vi "DEMO_Queue.vi"() -> ()   [LabVIEW 2018]
uses:
  DataPacker/DataStructures/GEM_BANK_CLUSTER_typedef.ctl
  DataPacker/DataStructures/GEM_DATA_cluster_typedef.ctl
  74751eb5-3986-46dd-b866-627731c09b6a.vi
  26fe34b5-c06c-455e-b018-4450bbc8faa2.vi
  74751eb5-3986-46dd-b866-627731c09b6a.vi/85c5be8d-80e5-4349-a72a-c74fdeb0c9bb.vi
  26fe34b5-c06c-455e-b018-4450bbc8faa2.vi/8747a64a-e124-4754-8124-08412923ccb0.vi
panel:
  in  "Request Debug Mode":bool
  in  "MIDAS Sever Port":u16=12345
  in  "MIDAS Server":string="my_midas_server.domain"
  out "RUNNO":i32
  in  "y":i32=2147483647
  in  "stop":bool
  out "# pending insert":i32
  out "# pending remove":i32
  out "# elements in queue":i32
  in  "Int entries to log":i32
  in  "IntState array":u32[](array[numeric])=[1, 2, 3, 4, 5, 6, 7, 8, 9, 10]
  in  "Entries to log":i32
  in  "Temperature array":dbl[](array[numeric])=[0.1, 0.2, 0.3, 0.4, 0.5, 0.6, 0.7, 0.8, 0.9, 1.0]
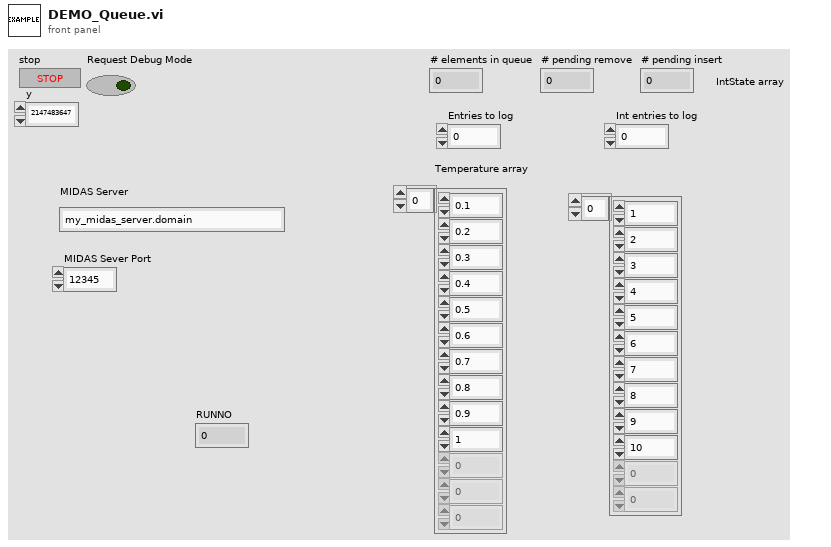
[diagram p1: front panel]
types:
  T1 = typedef "GEM_BANK_CLUSTER_typedef.ctl" = cluster{"Category":string, "Variable Name":string, "Equipment description":string, "History Settings":u16, "Period to update history plots":u16, "GEM_DATA Cluster":T2}
  T2 = typedef "GEM_DATA_cluster_typedef.ctl" = cluster{"DataType":string, "Formatted Data":u8[], "data byte order (Little Endian prefered)":enum16{"big-endian, network order", "native, host order", "little-endian"}}
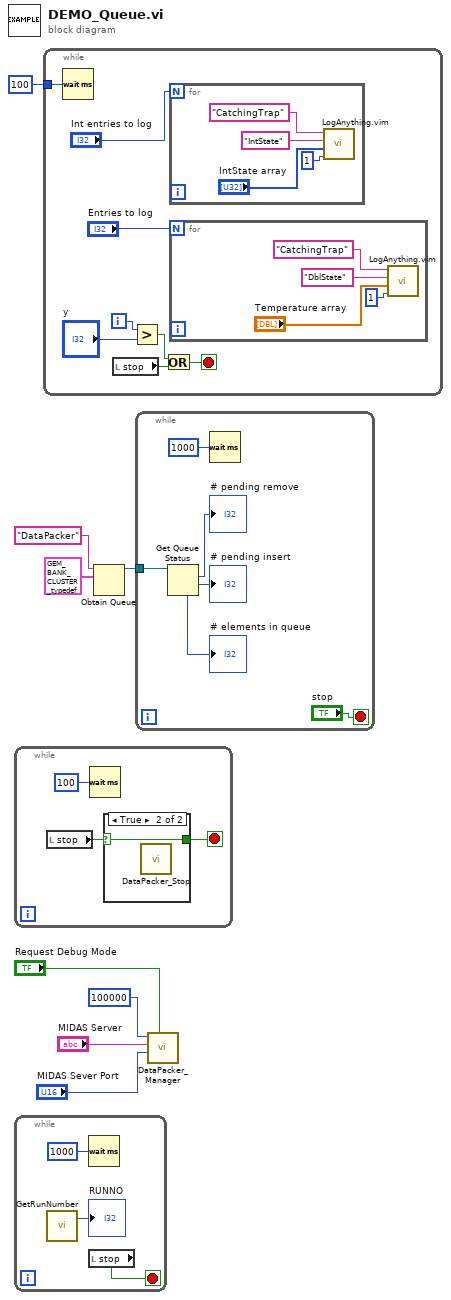
[diagram p0: block diagram]
diagram:
  n1 = while {
    stop <- w10 stop-if-true
    n2 = local read "stop"() -> (w9:bool)
    n3 = Wait (ms)(milliseconds to wait=u32 100) -> ()  [unwired: 1 out]
    n4 = case shown="True" w9 {
      selector: w9 -> [w12 w13]
      tunnel: [w12 w13] -> w10
      frame False {
      }
      frame True {
        n5 = call "DataPacker_Stop.vi"() -> ()  [unwired: 12 in]
      }
    }
  }
  n6 = while {
    stop <- w14 stop-if-true
    n7 = call "GetRunNumber.vi"() -> ("RunNumber"=→"RUNNO":i32)  [unwired: 2 in, 1 out]
    n8 = Wait (ms)(milliseconds to wait=u32 1000) -> ()  [unwired: 1 out]
    n9 = local read "stop"() -> (w14:bool)
  }
  n10 = while {
    tunnel: i64 100 ("Period") -> [w17]
    i -> [w18]
    stop <- w19 stop-if-true
    n11 = Wait (ms)(milliseconds to wait=w17) -> ()  [unwired: 1 out]
    n12 = local read "stop"() -> (w20:bool)
    n13 = Greater?(x=w18, y="y") -> (0:w21:bool)
    n14 = Or(x=w21, y=w20) -> (x .or. y?=w19:bool)
    n15 = for {
      N: "Int entries to log" -> [_]
      n16 = call "LogAnything.vim"("Period to update history plots (seconds)\nUnset (65535) = Use MIDAS default in ODB\n0 = Record but do not put in histories"=1 ("Rate to update history plots"), "Array"="IntState array", "Var Name"="IntState", "Category"="CatchingTrap") -> ()  [unwired: 3 in, 1 out]
    }
    n17 = for {
      N: "Entries to log" -> [_]
      n18 = call "LogAnything.vim"("Period to update history plots (seconds)\nUnset (65535) = Use MIDAS default in ODB\n0 = Record but do not put in histories"=1 ("Rate to update history plots"), "Array"="Temperature array", "Var Name"="DblState", "Category"="CatchingTrap") -> ()  [unwired: 3 in, 1 out]
    }
  }
  n19 = Obtain Queue(name (unnamed)="DataPacker", element data type=T1 {"Category"="", "Variable Name"="", "Equipment description"="", "History Settings"=0, "Period to update history plots"=0, "GEM_DATA Cluster"={"DataType"="", "Formatted Data"=[], "data byte order (Little Endian prefered)"=enum."big-endian, network order"}} ("output cluster")) -> (queue out=w7:refnum<queue>)  [unwired: 3 in, 2 out]
  n20 = while {
    tunnel: w7 -> [w38]
    stop <- "stop" stop-if-true
    n21 = Get Queue Status(queue=w38) -> (# pending remove=→"# pending remove":i32, # pending insert=→"# pending insert":i32, # elements in queue=→"# elements in queue":i32)  [unwired: 2 in, 5 out]
    n22 = Wait (ms)(milliseconds to wait=u32 1000) -> ()  [unwired: 1 out]
  }
  n23 = call "DataPacker_Manager.vi"("Request Debug Mode"="Request Debug Mode", "MIDAS Sever Port"="MIDAS Sever Port", "MIDAS Server"="MIDAS Server", "Override Max Event size (Data rate kb/s). Use MIDAS Default = 0"=u32 100000) -> ()  [unwired: 8 in]
